vi "Cochlear Function Test Suite.vi"() -> ()   [LabVIEW 2020]
uses:
  <vilib>/Utility/miscctls.llb/LVStringsAndValuesArrayTypeDef_U16.ctl
  CFTS VIs/CFTS-Experiment State.ctl
  CFTS VIs/CFTS-Options.ctl
  epl-vi-lib/Utility VIs/Error Handling VIs/Error-Library Action.ctl
  84bd467b-581b-4394-aac2-b4c4495df025.vi
  0e21acf6-e387-4aab-a16d-d10ed5c33526.vi
  epl-vi-lib/Utility VIs/File IO VIs/Read Write Anything/Read Anything.vi
  CFTS VIs/CFTS-Globals.vi
  <vilib>/Utility/config.llb/Open Config Data.vi
  <vilib>/Utility/config.llb/Get Key Names.vi
  <vilib>/Utility/config.llb/Read Key.vi
  <vilib>/Utility/config.llb/Read Key (String).vi
  epl-vi-lib/Utility VIs/Array Manipulation VIs/String Array to Comma Separated String.vi
  <vilib>/Utility/config.llb/Close Config Data.vi
panel:
  out "Debug":string="DEBUG"
  in  "Fast ABR":bool caption="Boolean"
  in  "Freefield":bool
  in  "ID":cluster{"Experimenter":string, "Number":u32} caption="Setup Options"
  in  "Other OAE":u16(ring) items=["Other OAE", "SFOAE", "SOAE"]
  in  "Undo":bool
  in  "Apply":bool
  in  "RW":u16(ring) items=["RW", "RW Noise", "PSTR"]
  in  "Other ABR":u16(ring) items=["Other ABR", "Masked ABR", "Fast ABR"]
  in  "Vitals":bool
  in  "Left":u16(ring) items=["---", "", "Bose", "Dummy", "DummyEA3A_ProbeTube.CALIB", "ER10C_1.25in", "ER10C_2in", "ER10C_3in", "ER10X", "ER10XProbeA", "ER10XProbeB", "Flat", "SN44_SU", "Speaker"]
  in  "Right":u16(ring) items=["---", "", "Bose", "Dummy", "DummyEA3A_ProbeTube.CALIB", "ER10C_1.25in", "ER10C_2in", "ER10C_3in", "ER10X", "ER10XProbeA", "ER10XProbeB", "Flat", "SN44_SU", "Speaker"]
  in  "CAP FM":bool caption="Boolean"
  in  "Options":bool
  in  "Help":bool
  in  "DP analysis":bool caption="Boolean"
  in  "Exposure":bool caption="Boolean"
  in  "System Test":bool
  in  "VsEP":bool caption="Boolean"
  out "VsEP Run#":i16
  in  "Connections":bool
  in  "VsEP Cal":bool
  in  "CAPTH":bool caption="Boolean"
  out "DP Run#":i16
  out "ABR Run#":i16
  out "CAP Run #":i16
  out "Data Folder":path
  in  "ABR":bool caption="Boolean"
  in  "DP I/O":bool caption="Boolean"
  in  "In-ear":bool
  in  "Calibrate probe tube":bool
  in  "Quit":bool caption="Boolean"
  # "Cochlear Function Test Suite"
  # "Calibration"
  # "Measurements"
  # "Acoustic Systems"
  # "CTRL-A toggles advanced menu"
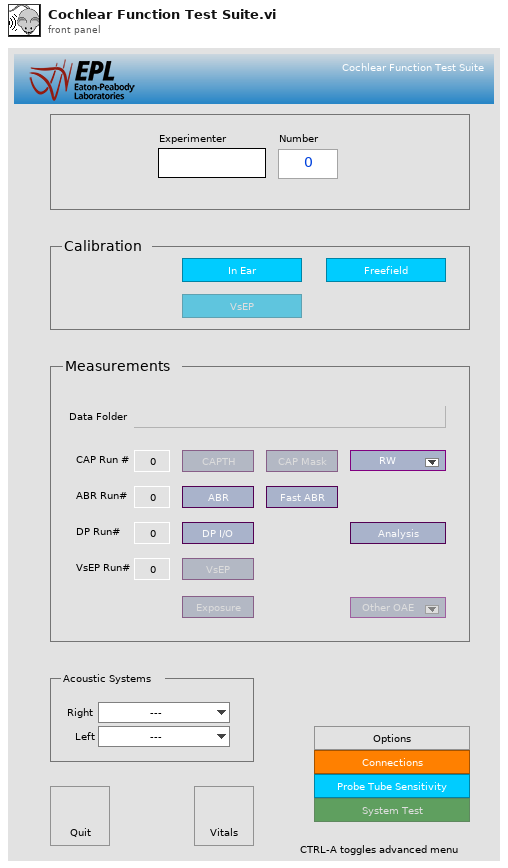
[diagram p1: front panel]
types:
  T1 = typedef "Error-Library Action.ctl" = enum16{"NONE", "Register", "Read"}
  T2 = typedef "CFTS-Options.ctl" = cluster{"Rig ID":string, "Acoustic System IDs":cluster{"Right":string, "Left":string}, "Extension":string, "Advanced users":string[], "All advanced":bool, "Run vitals":bool, "hash":string, "Allow nonEPL":bool, "NonEPL":string[], "Data root":path}
  T3 = typedef "CFTS-Experiment State.ctl" = cluster{"Experimenter":string, "Number":u32, "Right":string, "Left":string, "Data Folder":path, "Version":string, "End Exposure Time":dbl, "Exposure Duration":string, "Run #":cluster{"CAP":i32, "ABR":i32, "DP":i32, "VsEP":i32, "SFOAE":i32}}
  T4 = enum8{"Enabled", "Disabled", "Disabled and Grayed Out"}
  T5 = enum16{"big-endian, network order", "native, host order", "little-endian"}
  T6 = typedef "LVStringsAndValuesArrayTypeDef_U16.ctl" = cluster{"String":string, "Value":u16}[]
  T7 = typedef "CM-Endpoint.ctl" = cluster{"Name":string, "Device":string}
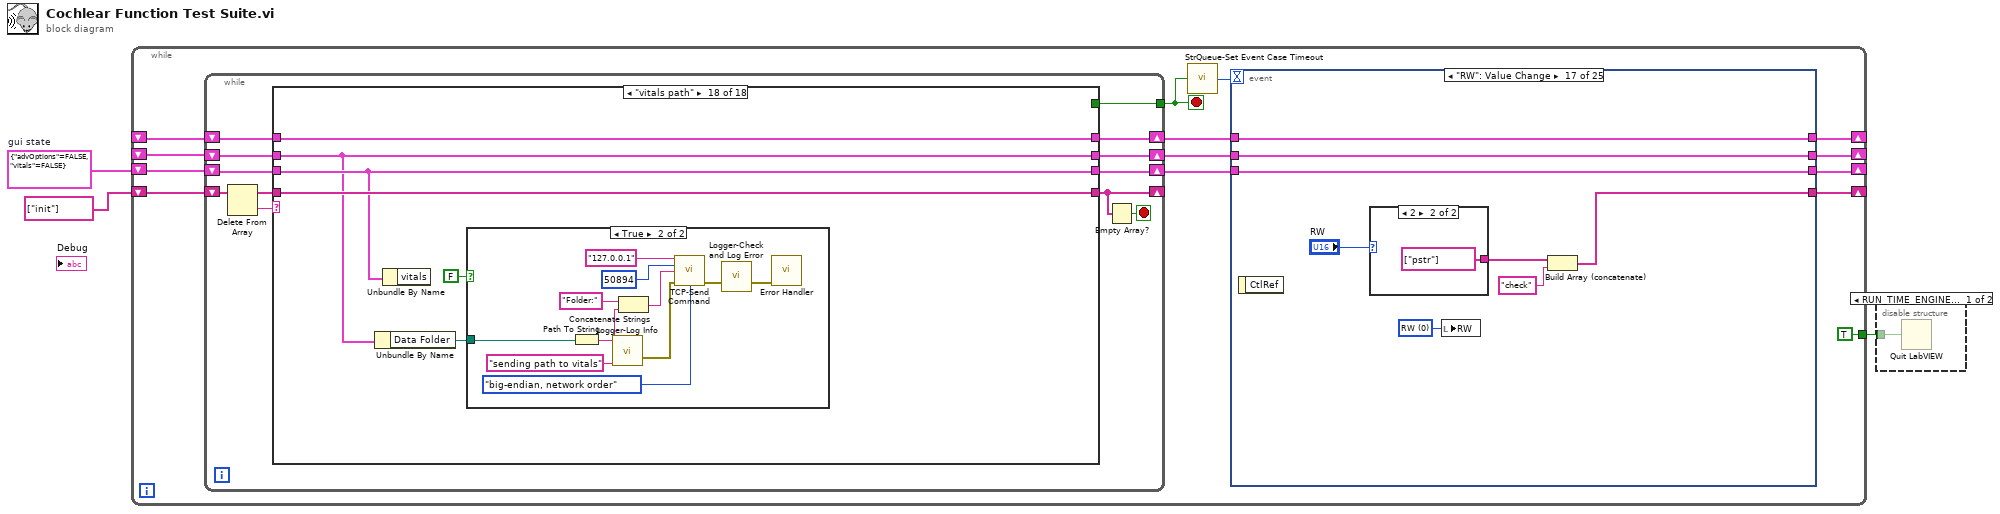
[diagram p0: block diagram]
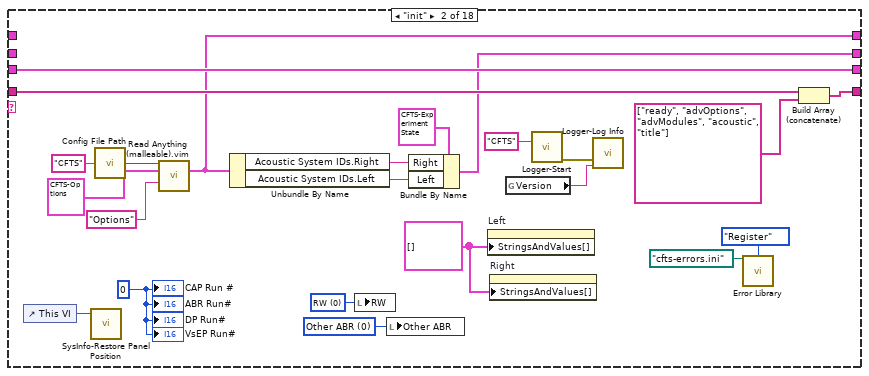
[diagram p3: hidden frame]
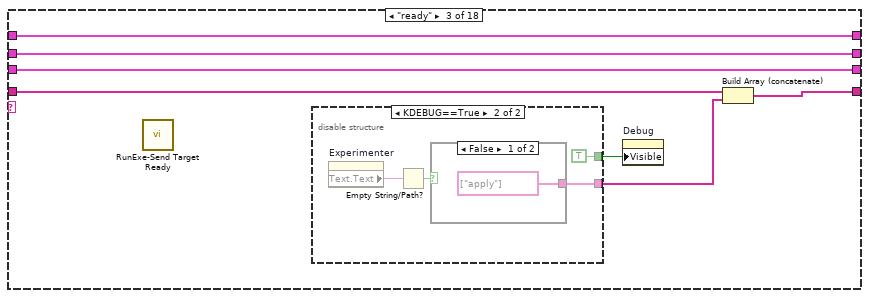
[diagram p4: hidden frame]
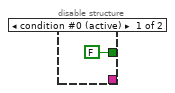
[diagram p5: hidden frame]
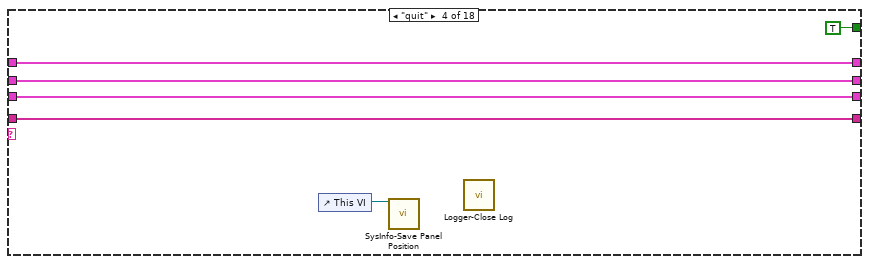
[diagram p7: hidden frame]
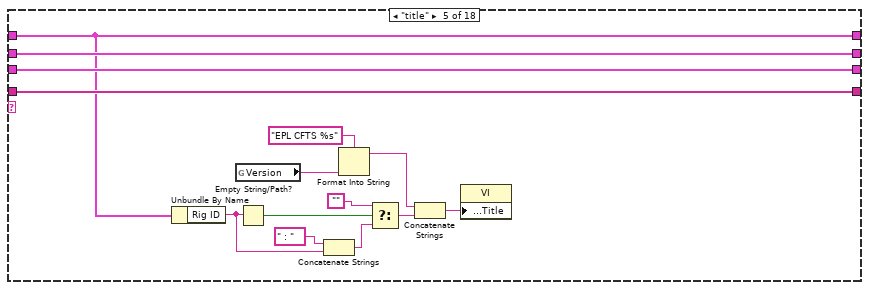
[diagram p8: hidden frame]
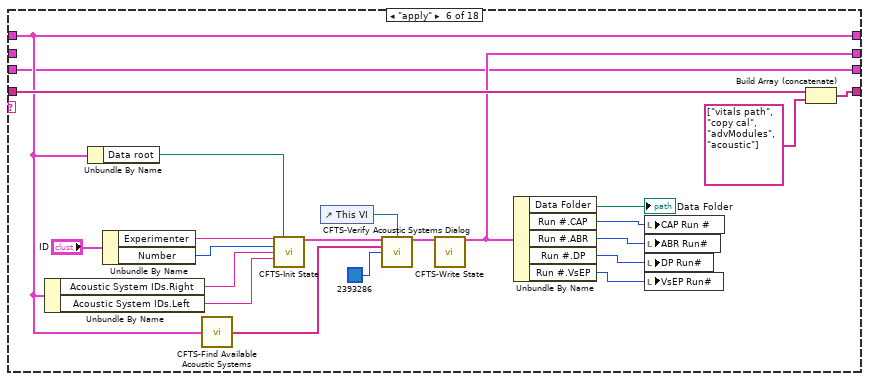
[diagram p9: hidden frame]
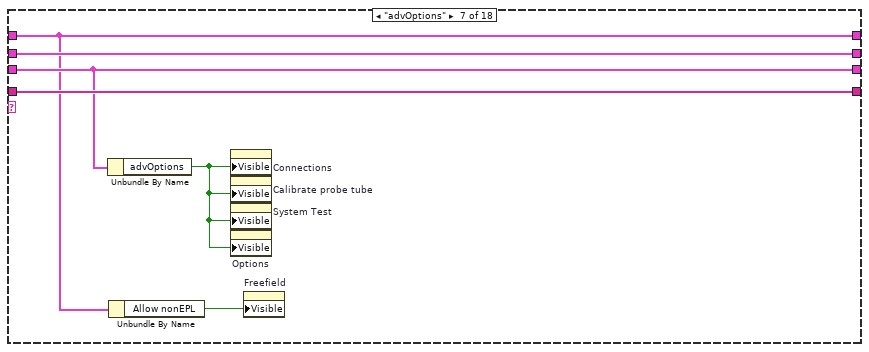
[diagram p10: hidden frame]
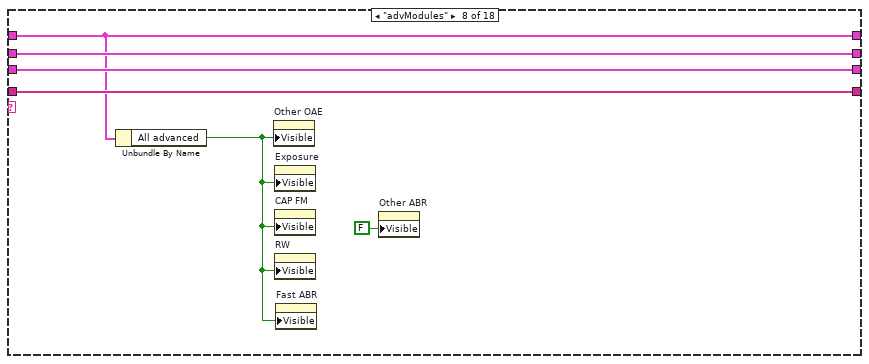
[diagram p11: hidden frame]
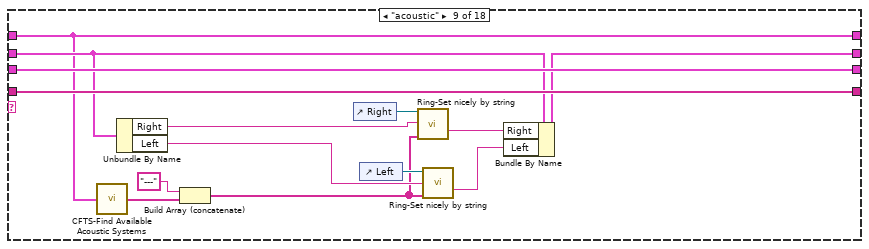
[diagram p12: hidden frame]
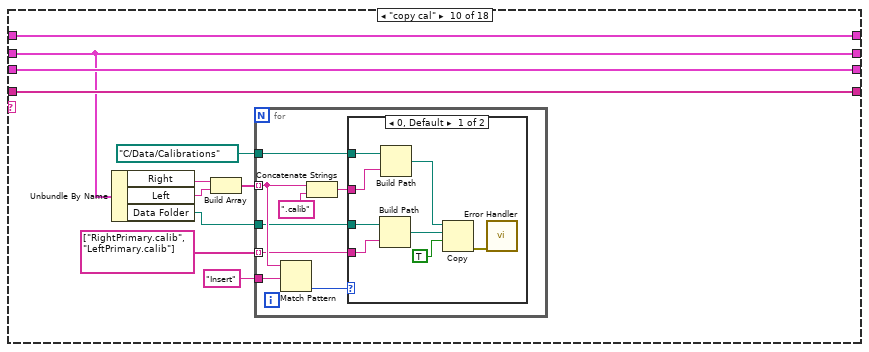
[diagram p13: hidden frame]
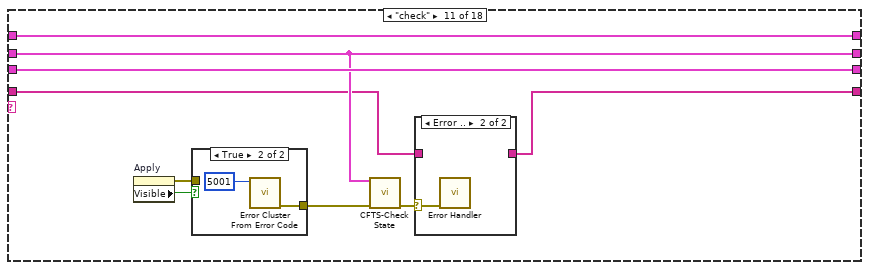
[diagram p15: hidden frame]
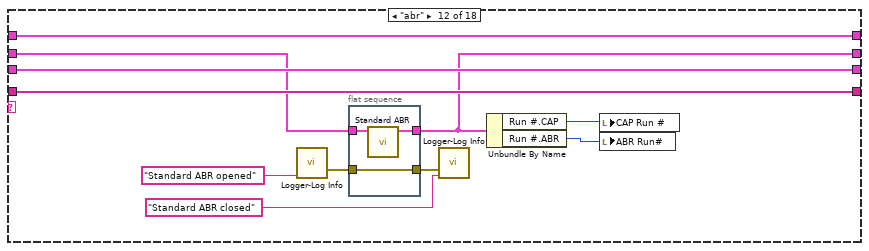
[diagram p18: hidden frame]
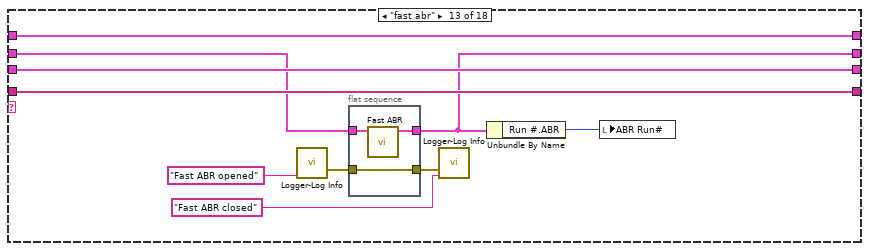
[diagram p19: hidden frame]
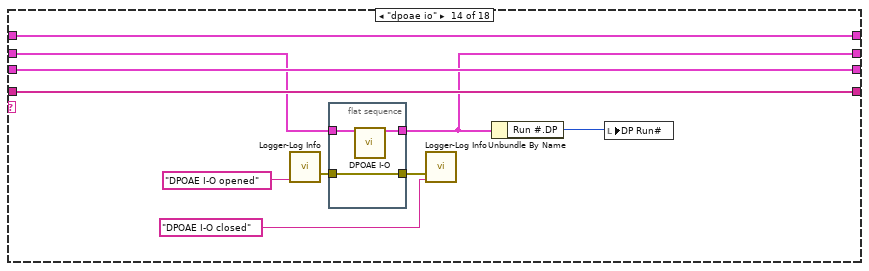
[diagram p20: hidden frame]
diagram:
  w2 = cluster{"advOptions":bool, "vitals":bool} {"advOptions"=FALSE, "vitals"=FALSE}  # gui state
  n1 = while {
    shift-right: [w12] -> _
    shift-left: _ -> [w16]
    tunnel: [TRUE] -> w3
    shift-right: [w11] -> _
    shift-left: w2 -> [w15]
    shift-right: [w7] -> _
    shift-left: string[] ["init"] ("Array") -> [w10]
    shift-right: [w6] -> _
    shift-left: _ -> [w4]
    stop <- w8 stop-if-true
    n2 = while {
      shift-right: [w26] -> _
      shift-left: w10 -> [w29]
      tunnel: [w24] -> w8
      shift-right: [w23] -> w14
      shift-left: w16 -> [w22]
      shift-right: [w20] -> w13
      shift-left: w15 -> [w21]
      shift-right: [w19] -> w5
      shift-left: w4 -> [w18]
      stop <- w25 stop-if-true
      n3 = Delete From Array(array=w29) -> (deleted portion=w27:string, array with subset deleted=w28:string[])  [unwired: 2 in]
      n4 = case shown="\"vitals path\"" w27 {
        tunnel: w28 -> [w33 w56 w63 w75 w89 w111 w117 w123 w137 w148 w166 w189 w202 w215 w227 w239 w258 w275]
        tunnel: [w33 w54 w58 w75 w89 w108 w117 w123 w137 w148 w165 w189 w202 w215 w227 w239 w244 w275] -> w26
        tunnel: [_ _ _ TRUE _ _ _ _ _ _ _ _ _ _ _ _ _ _] -> w24
        tunnel: [w32 w52 w62 w73 w88 w93 w116 w122 w128 w146 w168 w184 w198 w211 w224 w236 w248 w272] -> w23
        tunnel: w22 -> [w32 _ w62 w73 w88 _ w116 w122 w135 w146 w168 w183 w197 w210 w223 w236 w248 w272]
        tunnel: w21 -> [w31 w55 w61 w72 w87 w90 w115 w121 w136 w147 w173 w188 w201 w214 w226 w238 w257 w273]
        tunnel: [w31 w55 w61 w72 w87 w90 w115 w121 w136 w147 w173 w188 w201 w214 w226 w238 w245 w273] -> w20
        tunnel: [w30 w53 w60 w71 w80 w92 w113 w120 w125 w138 w172 w187 w200 w213 w225 w237 w256 w274] -> w19
        tunnel: w18 -> [w30 _ w60 w71 w80 w92 w113 w120 w125 w138 w172 w187 w200 w213 w225 w237 w256 w274]
        frame "", Default {
        }
        frame "init" {
          w48 = T6 [] ("Strings And Values []")
          w49 = i16 0 ("CAP RUN #")
          w51 = u16 0 items=["RW", "RW Noise", "PSTR"] ("RW")
          w50 = u16 0 items=["Other ABR", "Mask ABR", "Fast ABR"] ("Other ABR")
          n5 = control-ref of="This VI"() -> (w42:refnum<vi>)
          n6 = call "SysInfo-Restore Panel Position.vi"("VI Refnum"=w42) -> ()  [unwired: 12 in, 3 out]
          n7 = call "Config File Path.vi"("AppName"="CFTS") -> ("Default config file name"=w46:path)
          n8 = call "Read Anything (malleable).vim"("Config file path"=w46, "Options in"=T2 {"Rig ID"="", "Acoustic System IDs"={"Right"="", "Left"=""}, "Extension"=".tsv", "Advanced users"=[], "All advanced"=FALSE, "Run vitals"=FALSE, "hash"="", "Allow nonEPL"=FALSE, "NonEPL"=[], "Data root"=path ""} ("Options"), "Section"="Options") -> ("Options out"=w53:T2)  [unwired: 9 in, 3 out]
          n9 = Unbundle By Name(w53) -> ("Acoustic System IDs.Right"=w40:string, "Acoustic System IDs.Left"=w39:string)
          n10 = local write "RW"(w51) -> ()
          n11 = local write "Other ABR"(w50) -> ()
          n12 = Bundle By Name(cluster=T3 {"Experimenter"="", "Number"=0, "Right"="", "Left"="", "Data Folder"=path "", "Version"="", "End Exposure Time"=0.0, "Exposure Duration"="", "Run #"={"CAP"=0, "ABR"=0, "DP"=0, "VsEP"=0, "SFOAE"=0}} ("State"), "Right"=w40, "Left"=w39) -> (w52:T3)
          n13 = property on="Left" class="Ring (strict)"("StringsAndValues[]"=w48) -> ()  [unwired: 2 in, 2 out]
          n14 = property on="Right" class="Ring (strict)"("StringsAndValues[]"=w48) -> ()  [unwired: 2 in, 2 out]
          n15 = global read "CFTS-Globals.vi" "Version"() -> (w34:string)
          n16 = call "Logger-Start.vi"("Name"="CFTS") -> ("error out"=w35:errorcluster)  [unwired: 14 in]
          n17 = call "Logger-Log Info.vi"("error in (no error)"=w35, "Message"=w34) -> ()  [unwired: 13 in, 1 out]
          n18 = call "Error Library.vi"("Path"=path "cfts-errors.ini", "action"=Error-Library_Action."Register") -> ()  [unwired: 11 in, 3 out]
          n19 = Build Array (concatenate)(w56, string[] ["ready", "advOptions", "advModules", "acoustic", "title"]) -> (w54:string[])
          "CAP Run #" <- w49
          "ABR Run#" <- w49
          "DP Run#" <- w49
          "VsEP Run#" <- w49
        }
        frame "ready" {
          n20 = call "RunExe-Send Target Ready.vi"() -> ()  [unwired: 15 in, 1 out]
          n21 = disable-structure shown="KDEBUG==True" {
            disable-tunnel: [FALSE TRUE] -> w59
            disable-tunnel: [_ w68] -> w57
            frame condition #0 (active) {
            }
            frame condition #1 {
              n22 = property on="Experimenter" class="Str"() -> ("Text.Text"=w67:string)  [unwired: 2 in, 2 out]
              n23 = Empty String/Path?(string/path=w67) -> (empty?=w66:bool)
              n24 = case shown="False" w66 {
                tunnel: [string[] ["apply"] _] -> w68
                frame False {
                }
                frame True {
                }
              }
            }
          }
          n25 = property on="Debug" class="Str"("Visible"=w59) -> ()  [unwired: 2 in, 2 out]
          n26 = Build Array (concatenate)(w63, w57) -> (w58:string[])
        }
        frame "quit" {
          n27 = control-ref of="This VI"() -> (w70:refnum<vi>)
          n28 = call "SysInfo-Save Panel Position.vi"("VI Refnum"=w70) -> ()  [unwired: 14 in, 1 out]
          n29 = call "Logger-Close Log.vi"() -> ()  [unwired: 15 in, 1 out]
        }
        frame "title" {
          n30 = Unbundle By Name(w80) -> ("Rig ID"=w78:string)
          n31 = global read "CFTS-Globals.vi" "Version"() -> (w81:string)
          n32 = Empty String/Path?(string/path=w78) -> (empty?=w79:bool)
          n33 = Concatenate Strings(" : " ("string"), w78) -> (w77:string)
          n34 = Format Into String(format string="EPL CFTS %s" ("string"), w81) -> (resulting string=w83:string)  [unwired: 2 in, 1 out]
          n35 = Select(t="", s=w79, f=w77) -> (s? t:f=w86:string)
          n36 = Concatenate Strings(w83, w86) -> (w84:string)
          n37 = property class="VI"("Front Panel.Title"=w84) -> ()  [unwired: 2 in, 2 out]
        }
        frame "apply" {
          n38 = Unbundle By Name(w92) -> ("Acoustic System IDs.Right"=w100:string, "Acoustic System IDs.Left"=w99:string)
          n39 = Unbundle By Name(w92) -> ("Data root"=w91:path)
          n40 = Unbundle By Name("ID") -> ("Experimenter"=w104:string, "Number"=w103:u32)
          n41 = call "CFTS-Find Available Acoustic Systems.vi"("Options"=w92) -> ("Acoustic Systems"=w102:string[])  [unwired: 14 in]
          n42 = call "CFTS-Init State.vi"("Experimenter"=w104, "Root folder"=w91, "Num"=w103, "Right"=w100, "Left"=w99) -> ("State (out)"=w101:T3)  [unwired: 9 in, 1 out]
          n43 = control-ref of="This VI"() -> (w109:refnum<vi>)
          n44 = call "CFTS-Verify Acoustic Systems Dialog.vi"("Expt State"=w101, "center on"=w109, "Acoustic Systems"=w102, "color"=u32 2393286) -> ("Cluster out"=w94:T3)  [unwired: 10 in, 1 out]
          n45 = call "CFTS-Write State.vi"("State"=w94) -> ("State thru"=w93:T3)  [unwired: 13 in, 1 out]
          n46 = Unbundle By Name(w93) -> ("Data Folder"=→"Data Folder":path, "Run #.CAP"=w98:i32, "Run #.ABR"=w97:i32, "Run #.DP"=w96:i32, "Run #.VsEP"=w95:i32)
          n47 = local write "CAP Run #"(w98) -> ()
          n48 = local write "ABR Run#"(w97) -> ()
          n49 = local write "DP Run#"(w96) -> ()
          n50 = local write "VsEP Run#"(w95) -> ()
          n51 = Build Array (concatenate)(w111, string[] ["vitals path", "copy cal", "advModules", "acoustic"]) -> (w108:string[])
        }
        frame "advOptions" {
          n52 = Unbundle By Name(w115) -> ("advOptions"=w114:bool)
          n53 = Unbundle By Name(w113) -> ("Allow nonEPL"=w112:bool)
          n54 = property on="Connections" class="Bool"("Visible"=w114) -> ()  [unwired: 2 in, 2 out]
          n55 = property on="Calibrate probe tube" class="Bool"("Visible"=w114) -> ()  [unwired: 2 in, 2 out]
          n56 = property on="System Test" class="Bool"("Visible"=w114) -> ()  [unwired: 2 in, 2 out]
          n57 = property on="Options" class="Bool"("Visible"=w114) -> ()  [unwired: 2 in, 2 out]
          n58 = property on="Freefield" class="Bool"("Visible"=w112) -> ()  [unwired: 2 in, 2 out]
        }
        frame "advModules" {
          n59 = Unbundle By Name(w120) -> ("All advanced"=w118:bool)
          n60 = property on="Other OAE" class="Ring (strict)"("Visible"=w118) -> ()  [unwired: 2 in, 2 out]
          n61 = property on="Exposure" class="Bool"("Visible"=w118) -> ()  [unwired: 2 in, 2 out]
          n62 = property on="CAP FM" class="Bool"("Visible"=w118) -> ()  [unwired: 2 in, 2 out]
          n63 = property on="RW" class="Ring (strict)"("Visible"=w118) -> ()  [unwired: 2 in, 2 out]
          n64 = property on="Fast ABR" class="Bool"("Visible"=w118) -> ()  [unwired: 2 in, 2 out]
          n65 = property on="Other ABR" class="Ring (strict)"("Visible"=FALSE) -> ()  [unwired: 2 in, 2 out]
        }
        frame "acoustic" {
          n66 = call "CFTS-Find Available Acoustic Systems.vi"("Options"=w125) -> ("Acoustic Systems"=w124:string[])  [unwired: 14 in]
          n67 = Unbundle By Name(w135) -> ("Right"=w131:string, "Left"=w132:string)
          n68 = Build Array (concatenate)("---", w124) -> (w129:string[])
          n69 = control-ref of="Right"() -> (w134:refnum<vi>)
          n70 = control-ref of="Left"() -> (w133:refnum<vi>)
          n71 = call "Ring-Set nicely by string.vi"("Ring in"=w134, "Device"=w131, "Strings []"=w129) -> ("Selection"=w127:string)  [unwired: 8 in, 4 out]
          n72 = call "Ring-Set nicely by string.vi"("Ring in"=w133, "Device"=w132, "Strings []"=w129) -> ("Selection"=w126:string)  [unwired: 8 in, 4 out]
          n73 = Bundle By Name(cluster=w135, "Right"=w127, "Left"=w126) -> (w128:T3)
        }
        frame "copy cal" {
          n74 = Unbundle By Name(w146) -> ("Right"=w145:string, "Left"=w144:string, "Data Folder"=w140:path)
          n75 = Build Array(w145, w144) -> (w143:string[])
          n76 = for {
            tunnel: w143 -> [w154] mode=indexing
            tunnel: "Insert" ("regular expression") -> [w156]
            tunnel: path "C:/Data/Calibrations" ("path") -> [w151]
            tunnel: w140 -> [w150]
            tunnel: string[] ["RightPrimary.calib", "LeftPrimary.calib"] ("regular expression") -> [w149] mode=indexing
            n77 = Match Pattern(string=w154, regular expression=w156) -> (offset past match=w155:i32)  [unwired: 1 in, 3 out]
            n78 = Concatenate Strings(w154, ".calib") -> (w152:string)
            n79 = case shown="0, Default" w155 {
              tunnel: w152 -> [w161 _]
              tunnel: w151 -> [w162 _]
              tunnel: w150 -> [w159 _]
              tunnel: w149 -> [w158 _]
              frame 0, Default {
                n80 = Build Path(base path=w159, name or relative path=w158) -> (appended path=w164:path)
                n81 = Build Path(base path=w162, name or relative path=w161) -> (appended path=w160:path)
                n82 = Copy(9:TRUE ("overwrite (F)"), 10:w164, 11:w160) -> (0:w163:errorcluster)  [unwired: 2 in, 2 out]
                n83 = call "Error Handler.vi"("error in (no error)"=w163) -> ()  [unwired: 12 in, 3 out]
              }
              frame -1 {
              }
            }
          }
        }
        frame "check" {
          n84 = property on="Apply" class="Bool"() -> (error out=w170:errorcluster, "Visible"=w169:bool)  [unwired: 2 in, 1 out]
          n85 = case shown="True" w169 {
            tunnel: w170 -> [w176 _]
            tunnel: [w176 w177] -> w171
            frame False {
            }
            frame True {
              n86 = call <vilib>:"Error Cluster From Error Code.vi"("error code (0)"=5001) -> ("error out"=w177:errorcluster)  [unwired: 8 in]
            }
          }
          n87 = call "CFTS-Check State.vi"("Expt State"=w168, "error in (no error)"=w171) -> ("error out"=w167:errorcluster)  [unwired: 13 in]
          n88 = case shown="Error .." w167 {
            selector: w167 -> [_ w175]
            tunnel: w166 -> [w174 _]
            tunnel: [w174 _] -> w165
            frame No Error {
            }
            frame Error {
              n89 = call "Error Handler.vi"("error in (no error)"=w175) -> ()  [unwired: 12 in, 3 out]
            }
          }
        }
        frame "abr" {
          n90 = call "Logger-Log Info.vi"("Message"="Standard ABR opened" ("message")) -> ("error out"=w181:errorcluster)  [unwired: 14 in]
          n91 = flat-sequence {
            tunnel: [w192] -> w184
            tunnel: w183 -> [w191]
            tunnel: w181 -> [w190]
            tunnel: [w190] -> w180
            frame #0 {
              n92 = call "Standard ABR.vi"("State (in)"=w191) -> ("State"=w192:T3)  [unwired: 10 in]
            }
          }
          n93 = call "Logger-Log Info.vi"("error in (no error)"=w180, "Message"="Standard ABR closed" ("message")) -> ()  [unwired: 13 in, 1 out]
          n94 = Unbundle By Name(w184) -> ("Run #.CAP"=w186:i32, "Run #.ABR"=w185:i32)
          n95 = local write "CAP Run #"(w186) -> ()
          n96 = local write "ABR Run#"(w185) -> ()
        }
        frame "fast abr" {
          n97 = call "Logger-Log Info.vi"("Message"="Fast ABR opened" ("message")) -> ("error out"=w195:errorcluster)  [unwired: 14 in]
          n98 = flat-sequence {
            tunnel: [w205] -> w198
            tunnel: w197 -> [w204]
            tunnel: w195 -> [w203]
            tunnel: [w203] -> w194
            frame #0 {
              n99 = call "Fast ABR.vi"("State (in)"=w204) -> ("State (out)"=w205:T3)  [unwired: 10 in]
            }
          }
          n100 = call "Logger-Log Info.vi"("error in (no error)"=w194, "Message"="Fast ABR closed" ("message")) -> ()  [unwired: 13 in, 1 out]
          n101 = Unbundle By Name(w198) -> ("Run #.ABR"=w199:i32)
          n102 = local write "ABR Run#"(w199) -> ()
        }
        frame "dpoae io" {
          n103 = call "Logger-Log Info.vi"("Message"="DPOAE I-O opened" ("message")) -> ("error out"=w208:errorcluster)  [unwired: 14 in]
          n104 = flat-sequence {
            tunnel: [w218] -> w211
            tunnel: w210 -> [w217]
            tunnel: w208 -> [w216]
            tunnel: [w216] -> w207
            frame #0 {
              n105 = call "DPOAE I-O.vi"("State in"=w217) -> ("State out"=w218:T3)  [unwired: 14 in]
            }
          }
          n106 = call "Logger-Log Info.vi"("error in (no error)"=w207, "Message"="DPOAE I-O closed" ("message")) -> ()  [unwired: 13 in, 1 out]
          n107 = Unbundle By Name(w211) -> ("Run #.DP"=w212:i32)
          n108 = local write "DP Run#"(w212) -> ()
        }
        frame "pstr" {
          n109 = call "Logger-Log Info.vi"("Message"="PSTR opened" ("message")) -> ("error out"=w221:errorcluster)  [unwired: 14 in]
          n110 = flat-sequence {
            tunnel: [w230] -> w224
            tunnel: w223 -> [w229]
            tunnel: w221 -> [w228]
            tunnel: [w228] -> w220
            frame #0 {
              n111 = call "PSTR Controller.vi"("Expt State (in)"=w229) -> ("Expt State"=w230:T3)  [unwired: 10 in]
            }
          }
          n112 = call "Logger-Log Info.vi"("error in (no error)"=w220, "Message"="PSTR closed" ("message")) -> ()  [unwired: 13 in, 1 out]
        }
        frame "dp analysis" {
          n113 = Unbundle By Name(w236) -> ("Data Folder"=w235:path)
          n114 = call "Logger-Log Info.vi"("Message"="DPOAE analysis panel opened" ("message")) -> ("error out"=w231:errorcluster)  [unwired: 14 in]
          n115 = flat-sequence {
            tunnel: w235 -> [w241]
            tunnel: [w240] -> w232
            tunnel: w231 -> [w240]
            frame #0 {
              n116 = call "DPOAE Analysis Panel.vi"("Data folder in"=w241) -> ()  [unwired: 11 in]
            }
          }
          n117 = call "Logger-Log Info.vi"("error in (no error)"=w232, "Message"="DPOAE analysis panel closed" ("message")) -> ()  [unwired: 13 in, 1 out]
        }
        frame "vitals" {
          n118 = Unbundle By Name(w248) -> ("Experimenter"=w247:string)
          n119 = Empty String/Path?(string/path=w247) -> (empty?=w246:bool)
          n120 = call "CFTS-Open Vitals Monitor.vi"() -> ("error out"=w255:errorcluster)  [unwired: 15 in]
          n121 = call "Logger-Log Info.vi"("Message"="Opening vitals" ("message")) -> ("error out"=w250:errorcluster)  [unwired: 14 in]
          n122 = case shown="No Error" w255 {
            selector: w255 -> [_ w269]
            tunnel: [w264 w268] -> w254
            tunnel: T4."Enabled" ("Disabled") -> [w264 w268]
            tunnel: [w263 w267] -> w251
            tunnel: w250 -> [w263 w267]
            tunnel: ["Vitals opened" ("message") "Failed to open vitals" ("message")] -> w249
            tunnel: w246 -> [w261 _]
            tunnel: [w260 _] -> w243
            tunnel: [TRUE _] -> w242
            frame No Error {
              n123 = case shown="False" w261 {
                tunnel: [string[] ["vitals path"] _] -> w260
                frame False {
                }
                frame True {
                }
              }
            }
            frame Error {
              n124 = call "Error Handler.vi"("error in (no error)"=w269) -> ()  [unwired: 12 in, 3 out]
            }
          }
          n125 = Bundle By Name(cluster=w257, "vitals"=w242) -> (w245:cluster{"advOptions":bool, "vitals":bool})
          n126 = property on="Vitals" class="Bool"("DisabledEnum"=w254) -> ()  [unwired: 2 in, 2 out]
          n127 = call "Logger-Log Info.vi"("error in (no error)"=w251, "Message"=w249) -> ()  [unwired: 13 in, 1 out]
          n128 = Build Array (concatenate)(w258, w243) -> (w244:string[])
        }
        frame "vitals path" {
          n129 = Unbundle By Name(w272) -> ("Data Folder"=w271:path)
          n130 = Unbundle By Name(w273) -> ()  [unwired: 1 out]
          n131 = case shown="True" FALSE {
            tunnel: w271 -> [_ w282]
            frame False {
            }
            frame True {
              n132 = Path To String(path=w282) -> (string=w281:string)
              n133 = call "Logger-Log Info.vi"("Message"="sending path to vitals") -> ("error out"=w279:errorcluster)  [unwired: 14 in]
              n134 = Concatenate Strings("Folder:" ("Command"), w281) -> (w283:string)
              n135 = call "TCP-Send Command.vi"("PXI Address"="127.0.0.1", "Port"=50894, "Command"=w283, "error in (no error)"=w279, "byte order"=T5."big-endian, network order") -> ("error out"=w278:errorcluster)  [unwired: 10 in]
              n136 = call "Logger-Check and Log Error.vi"("error in (no error)"=w278) -> ("error out"=w277:errorcluster)  [unwired: 14 in]
              n137 = call "Error Handler.vi"("error in (no error)"=w277) -> ()  [unwired: 12 in, 3 out]
            }
          }
        }
      }
      n138 = Empty Array?(array=w26) -> (empty?=w25:bool)
    }
    n139 = call "StrQueue-Set Event Case Timeout.vi"("Quit"=w8) -> ("timeout"=w9:i32)  [unwired: 14 in]
    n140 = event shown="[16] \"RW\": Value Change" {
      selector: _ -> [_ _ _ _ _ _ _ _ _ _ _ _ _ _ _ _ _ _ _ _ _ _ _ _ _]
      dyn-events: _ -> [_ _ _ _ _ _ _ _ _ _ _ _ _ _ _ _ _ _ _ _ _ _ _ _ _]
      timeout: w9 -> [_ _ _ _ _ _ _ _ _ _ _ _ _ _ _ _ _ _ _ _ _ _ _ _ _]
      tunnel: w14 -> [w288 w293 w301 w335 w339 w347 w351 w358 w364 w379 w399 w403 w405 w409 w413 w418 w426 w435 w442 w453 w461 w472 w480 w485 w490]
      tunnel: [w288 w293 w301 w335 w339 w347 w351 w358 w363 w379 w399 w403 w405 w409 w413 w418 w426 w435 w442 w453 w461 w472 w480 w485 w490] -> w12
      tunnel: [_ string[] ["quit"] w299 string[] ["quit"] _ _ string[] ["apply"] _ _ _ _ _ string[] ["abr", "check"] string[] ["fast abr", "check"] string[] ["dpoae io", "check"] _ w419 w430 _ string[] ["dp analysis"] w455 _ string[] ["acoustic"] _ string[] ["vitals"]] -> w7
      tunnel: [w289 w291 w300 w333 w337 w345 w350 w355 w360 w381 w400 w402 w407 w411 w415 w417 w425 w434 w441 w452 w460 w471 w482 w484 w489] -> w11
      tunnel: w13 -> [w289 w291 w297 w333 w337 w345 w350 w355 w360 w381 w400 w402 w407 w411 w415 w417 w425 w434 w441 w452 w460 w471 w482 w484 w489]
      tunnel: [w287 w290 w296 w332 w336 w344 w348 w354 w359 w380 w396 w401 w406 w410 w414 w416 w423 w433 w439 w451 w456 w470 w481 w483 w488] -> w6
      tunnel: w5 -> [w287 w290 w296 w332 w336 w344 w348 w354 w359 w380 w396 w401 w406 w410 w414 w416 w423 w433 w439 w451 w457 w470 w481 w483 w488]
      event Timeout {
        n141 = event-data() -> ()  [unwired: 1 in, 1 out]
      }
      event Panel Close? {
        n142 = event-data() -> ()  [unwired: 1 in, 1 out]
        n143 = event-data("Discard?"=TRUE) -> ()  [unwired: 1 in, 1 out]
      }
      event Key Up {
        w305 = i16 30  # "A"
        n144 = event-data() -> ("ScanCode"=w306:i16, "PlatMods.Ctrl"=w303:bool)  [unwired: 1 in]
        n145 = Unbundle By Name(w297) -> ("advOptions"=w298:bool)
        n146 = Unbundle By Name(w296) -> ("hash"=w295:string)
        n147 = Equal?(x=w305, y=w306) -> (x = y?=w304:bool)
        n148 = And(x=w304, y=w303) -> (x .and. y?=w302:bool)
        n149 = case shown="True" w302 {
          tunnel: [w307 w312] -> w300
          tunnel: [_ w311] -> w299
          tunnel: w298 -> [_ w310]
          tunnel: w297 -> [w307 w309]
          tunnel: w295 -> [_ w308]
          frame False {
          }
          frame True {
            n150 = case shown="False" w310 {
              tunnel: [w315 w331] -> w312
              tunnel: [w313 string[] ["advOptions"]] -> w311
              tunnel: w309 -> [w316 w329]
              tunnel: w308 -> [w317 _]
              frame False {
                n151 = case shown="\"any\", Default" w317 {
                  selector: w317 -> [w320 _]
                  tunnel: [w318 TRUE] -> w314
                  frame "any", Default {
                    n152 = control-ref of="This VI"() -> (w321:refnum<vi>)
                    n153 = call "CFTS-Password Dialog.vi"("Parent VI"=w321) -> ("hash"=w319:string)  [unwired: 14 in]
                    n154 = Equal?(x=w320, y=w319) -> (x = y?=w318:bool)
                  }
                  frame "" {
                  }
                }
                n155 = case shown="True" w314 {
                  tunnel: w316 -> [w323 w327]
                  tunnel: [w323 w326] -> w315
                  tunnel: [_ string[] ["advOptions"]] -> w313
                  frame False {
                  }
                  frame True {
                    n156 = Bundle By Name(cluster=w327, "advOptions"=TRUE) -> (w326:cluster{"advOptions":bool, "vitals":bool})
                  }
                }
              }
              frame True {
                n157 = Bundle By Name(cluster=w329, "advOptions"=FALSE) -> (w331:cluster{"advOptions":bool, "vitals":bool})
              }
            }
          }
        }
      }
      event "Quit": Value Change {
        n158 = event-data() -> ()  [unwired: 1 in, 1 out]
      }
      event "Help": Value Change {
        n159 = event-data() -> ("NewVal"=w338:bool)  [unwired: 1 in]
        n160 = disable-structure shown="Disabled" {
          disable-tunnel: w338 -> [w340 _]
          frame Disabled {
            n161 = case shown="True" w340 {
              frame False {
              }
              frame True {
                n162 = call "Open Help Topic.vi"("Help file"="CFTS", "HelpId"=9) -> ("error out"=w342:errorcluster)  [unwired: 13 in]
                n163 = call "Error Handler.vi"("error in (no error)"=w342) -> ()  [unwired: 12 in, 3 out]
              }
            }
          }
          frame Enabled {
          }
        }
      }
      event "ID.Experimenter", "ID.Number": Value Change {
        w346 = TRUE ("Visible")
        n164 = event-data() -> ()  [unwired: 1 in, 1 out]
        n165 = property on="Undo" class="Bool"("Visible"=w346) -> ()  [unwired: 2 in, 2 out]
        n166 = property on="Apply" class="Bool"("Visible"=w346) -> ()  [unwired: 2 in, 2 out]
      }
      event "Apply": Value Change {
        w352 = FALSE
        n167 = event-data() -> ()  [unwired: 1 in, 1 out]
        n168 = property on="Apply" class="Bool"("Visible"=w352) -> (error out=w353:errorcluster)  [unwired: 2 in, 1 out]
        n169 = property on="Undo" class="Bool"(error in=w353, "Visible"=w352) -> ()  [unwired: 1 in, 2 out]
      }
      event "Undo": Value Change {
        w357 = FALSE
        n170 = event-data() -> ()  [unwired: 1 in, 1 out]
        n171 = property on="Apply" class="Bool"("Visible"=w357) -> (error out=w356:errorcluster)  [unwired: 2 in, 1 out]
        n172 = property on="Undo" class="Bool"(error in=w356, "Visible"=w357) -> ()  [unwired: 1 in, 2 out]
      }
      event "Right", "Left": Value Change {
        n173 = event-data() -> ()  [unwired: 1 in, 1 out]
        n174 = property on="Right" class="Ring (strict)"() -> ("RingText.Text"=w361:string)  [unwired: 2 in, 2 out]
        n175 = property on="Left" class="Ring (strict)"() -> ("RingText.Text"=w362:string)  [unwired: 2 in, 2 out]
        n176 = Bundle By Name(cluster=w364, "Right"=w361, "Left"=w362) -> (w363:T3)
      }
      event "In-ear": Value Change {
        n177 = event-data() -> ()  [unwired: 1 in, 1 out]
        n178 = Unbundle By Name(w379) -> ("Experimenter"=w378:string, "Data Folder"=w377:path, "Right"=w376:string, "Left"=w375:string)
        n179 = Build Array(w376, w375) -> (w373:string[])
        n180 = for {
          tunnel: path "C:/Data/Probe Tube Calibrations" -> [w386]
          tunnel: w373 -> [w384] mode=indexing
          tunnel: "_ProbeTube.calib" -> [w383]
          tunnel: [w382] -> w371 mode=indexing
          n181 = Concatenate Strings(w384, w383) -> (w385:string)
          n182 = Build Path(base path=w386, name or relative path=w385) -> (appended path=w382:path)
        }
        n183 = call "CFTS-Read Connections.vi"("Which"="Analog Outputs") -> ("endpoints"=w367:T7[])  [unwired: 13 in, 1 out]
        n184 = call "CFTS-Read Connections.vi"("Which"="Analog Inputs") -> ("endpoints"=w365:T7[])  [unwired: 13 in, 1 out]
        n185 = Index Array(array=w371) -> (element #1=w370:path, element #2=w369:path)  [unwired: 2 in]
        n186 = call "Calibrate In Ear.vi"("Data folder"=w377, "Experimenter"=w378, "Right PT"=w370, "Left PT"=w369, "Outputs"=w367, "Inputs"=w365) -> ()  [unwired: 10 in]
      }
      event "Freefield": Value Change {
        n187 = event-data() -> ()  [unwired: 1 in, 1 out]
        n188 = Unbundle By Name(w396) -> ("NonEPL"=w395:string[])
        n189 = call "Config File Path.vi"("AppName"="CFTS") -> ("Default config file name"=w389:path)
        n190 = call "Config File Path.vi"("AppName"="CFTS") -> ("Default config file name"=w392:path)
        n191 = call "CM-Read Configuration.vi"("Connection File Path"=w392, "Section"="Analog Outputs", "Outputs"=w395) -> ("Endpoints"=w394:T7[])  [unwired: 8 in, 4 out]
        n192 = call "CM-Endpoint Name To Device.vim"("Path"=w389, "IO Type"="Analog Inputs" ("Section"), "Names in"="Cal Mic") -> ("Devices"=w387:string)  [unwired: 9 in, 3 out]
        n193 = call "Freefield Calibration.vi"("Folder"=path "C:/Data/Calibrations", "Endpoints"=w394, "Mic device"=w387) -> ()  [unwired: 13 in]
      }
      event "VsEP Cal": Value Change {
        n194 = event-data() -> ()  [unwired: 1 in, 1 out]
      }
      event "ABR": Value Change {
        n195 = event-data() -> ()  [unwired: 1 in, 1 out]
      }
      event "Fast ABR": Value Change {
        n196 = event-data() -> ()  [unwired: 1 in, 1 out]
      }
      event "DP I/O": Value Change {
        n197 = event-data() -> ()  [unwired: 1 in, 1 out]
      }
      event "CAPTH", "VsEP", "Exposure", "CAP FM": Value Change {
        n198 = event-data() -> ()  [unwired: 1 in, 1 out]
      }
      event "RW": Value Change {
        w424 = u16 0 items=["RW", "RW Noise", "PSTR"] ("RW")
        n199 = event-data() -> ()  [unwired: 1 in, 1 out]
        n200 = case shown="2" "RW" {
          tunnel: [_ string[] ["pstr"]] -> w421
          frame 0, Default {
          }
          frame 2 {
          }
        }
        n201 = local write "RW"(w424) -> ()
        n202 = Build Array (concatenate)(w421, "check" ("String")) -> (w419:string[])
      }
      event "Other ABR": Value Change {
        w429 = u16 0 items=["Other ABR", "Masked ABR", "Fast ABR"] ("Other ABR")
        n203 = event-data() -> ("CtlRef"=w432:refnum<vi>)  [unwired: 1 in]
        n204 = property class="Ring (strict)"(reference=w432) -> ("RingText.Text"=w431:string)  [unwired: 1 in, 2 out]
        n205 = case shown="\"Fast ABR\"" w431 {
          tunnel: [_ string[] ["fast abr", "check"]] -> w430
          tunnel: [w436 w437] -> w428
          tunnel: w429 -> [w436 w437]
          frame Default {
          }
          frame "Fast ABR" {
          }
        }
        n206 = local write "Other ABR"(w428) -> ()
      }
      event "Other OAE": Value Change {
        w440 = u16 0 items=["Other OAE", "SFOAE", "SOAE"] ("Other OAE")
        n207 = event-data() -> ()  [unwired: 1 in, 1 out]
        n208 = property on="Apply" class="Bool"() -> (error out=w444:errorcluster, "Visible"=w445:bool)  [unwired: 2 in, 1 out]
        n209 = case shown="True" w445 {
          tunnel: w444 -> [w447 _]
          tunnel: [w447 w448] -> w443
          frame False {
          }
          frame True {
            n210 = call <vilib>:"Error Cluster From Error Code.vi"("error code (0)"=5001) -> ("error out"=w448:errorcluster)  [unwired: 8 in]
          }
        }
        n211 = call "CFTS-Check State.vi"("Expt State"=w442, "error in (no error)"=w443) -> ("error out"=w446:errorcluster)  [unwired: 13 in]
        n212 = local write "Other OAE"(w440) -> ()
        n213 = call "Error Handler.vi"("error in (no error)"=w446) -> ()  [unwired: 12 in, 3 out]
      }
      event "DP analysis": Value Change {
        n214 = event-data() -> ()  [unwired: 1 in, 1 out]
      }
      event "Options": Value Change {
        n215 = event-data() -> ()  [unwired: 1 in, 1 out]
        n216 = control-ref of="This VI"() -> (w454:refnum<vi>)
        n217 = call "CFTS-Options Dialog.vi"("Options in"=w457, "Parent VI"=w454) -> ("Options out"=w458:T2, "Cancelled?"=w459:bool)  [unwired: 12 in]
        n218 = case shown="False" w459 {
          tunnel: w458 -> [w464 _]
          tunnel: w457 -> [_ w468]
          tunnel: [w464 w468] -> w456
          tunnel: [w463 _] -> _
          tunnel: [string[] ["advModules", "acoustic", "title"] _] -> w455
          frame False {
            n219 = call "Config File Path.vi"("AppName"="CFTS") -> ("Default config file name"=w466:path)
            n220 = call "Write Anything.vi"("Section Name (Name of \"Anything\")"="Options" ("Section"), "Anything"=w464, "Path (dialog)"=w466) -> ("Error Out"=w463:errorcluster)  [unwired: 7 in, 1 out]
          }
          frame True {
          }
        }
      }
      event "Connections": Value Change {
        n221 = event-data() -> ()  [unwired: 1 in, 1 out]
        n222 = control-ref of="This VI"() -> (w469:refnum<vi>)
        n223 = call "CFTS-Connections Dialog.vi"("Parent VI"=w469) -> ()  [unwired: 15 in]
      }
      event "Calibrate probe tube": Value Change {
        n224 = event-data() -> ()  [unwired: 1 in, 1 out]
        n225 = Unbundle By Name(w480) -> ("Right"=w474:string, "Left"=w473:string)
        n226 = call "CFTS-Read Connections.vi"("Which"="Analog Outputs") -> ("endpoints"=w478:T7[])  [unwired: 13 in, 1 out]
        n227 = call "CFTS-Read Connections.vi"("Which"="Analog Inputs") -> ("endpoints"=w476:T7[])  [unwired: 13 in, 1 out]
        n228 = call "Calibrate Probe Tube.vi"("Right"=w474, "Left"=w473, "Outputs"=w478, "Inputs"=w476) -> ()  [unwired: 12 in]
      }
      event "System Test": Value Change {
        n229 = event-data() -> ()  [unwired: 1 in, 1 out]
      }
      event "Vitals": Value Change {
        n230 = event-data() -> ()  [unwired: 1 in, 1 out]
        n231 = property on="Vitals" class="Bool"("DisabledEnum"=T4."Disabled and Grayed Out" ("Disabled")) -> ()  [unwired: 2 in, 2 out]
      }
    }
  }
  n232 = disable-structure shown="RUN_TIME_ENGINE==True" {
    disable-tunnel: w3 -> [w491 _]
    frame condition #0 {
      n233 = Quit LabVIEW(quit? (T)=w491) -> ()
    }
    frame condition #1 (active) {
    }
  }
